vi "Initialize.vi"(8 "Error In":errorcluster, 11 "libssh2lv Shared Library":path=path "") -> (0 "Error Out":errorcluster, 3 "SSH":refnum<class "SSH.lvclass">)   [LabVIEW 2021, in "Field_RnD_Services_LIBSSH2_Toolkit.lvlib" / "SSH.lvclass"]
doc: "Initialize the underlying libssh2 library. This must be called, or executed, before using any other VIs in this toolkit. This typically initializes the cryptography library (OpenSSL), which is statically compiled with the libssh2lv shared library."
uses:
  220524-VNA RP FLAT.llb/SSH.lvclass
  220524-VNA RP FLAT.llb/SSH.lvclass/SSH.ctl
  220524-VNA RP FLAT.llb/Field_RnD_Services_LIBSSH2_Toolkit.lvlib
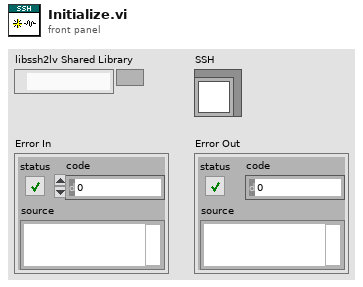
[diagram p1: front panel]
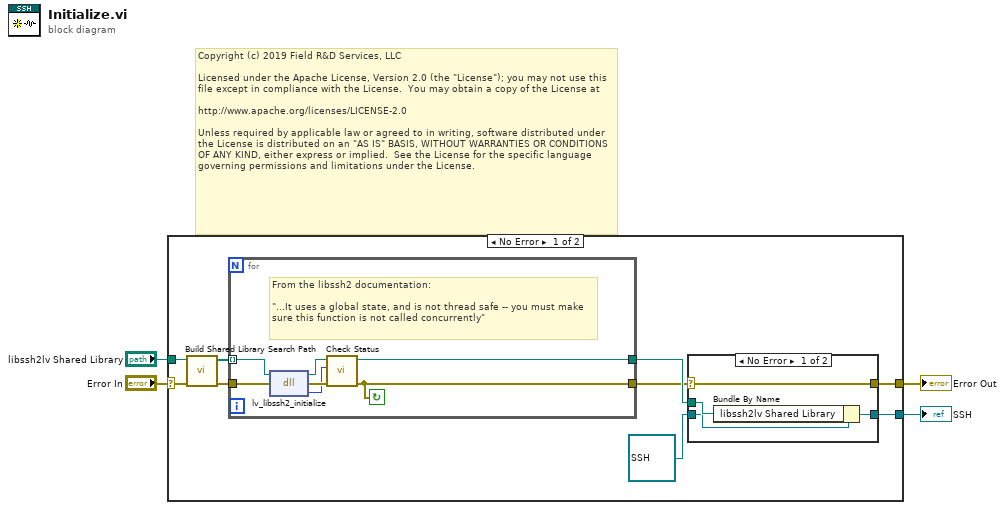
[diagram p0: block diagram]
diagram:
  # "Copyright (c) 2019 Field R&D Services, LLC\n\nLicensed under the Apache License, Version 2.0 (the \"License\"); you may not use this file except in compliance with the License.  You may obtain a copy of the License at\n\nhttp://www.apache.org/licenses/LICENSE-2.0\n\nUnless required by applicable law or agreed to in writing, software distributed under the License is distributed on an \"AS IS\" BASIS, WITHOUT WARRANTIES OR CONDITIONS OF ANY KIND, either express or implied.  See the License for the specific language governing permissions and limitations under the License."
  n1 = case shown="No Error" "Error In" {
    selector: "Error In" -> [w13 w27]
    tunnel: "libssh2lv Shared Library" -> [w12 _]
    tunnel: [w6 w27] -> w2
    tunnel: [w8 _] -> w1
    frame No Error {
      n2 = call "Build Shared Library Search Path.vi"("Error In"=w13, "libssh2lv Shared Library"=w12) -> ("Error Out"=w10:errorcluster, "Search Path"=w11:path[])  [unwired: 8 in]
      n3 = for {
        tunnel: w11 -> [w23] mode=indexing
        tunnel: w10 -> [w24]
        tunnel: [w26] -> w9
        tunnel: [w25] -> w7
        stop <- w25 continue-if-true
        # "From the libssh2 documentation:\n\n\"...It uses a global state, and is not thread safe -- you must make sure this function is not called concurrently\""
        n4 = dll-call lib="libssh2lv.*" fn="lv_libssh2_initialize"(path in=w23, error in=w24) -> (path out=w21:path, error out=w22:errorcluster, "return type"=w20:i32)  [unwired: 1 in]
        n5 = call "Check Status.vi"("Error In"=w22, "Status"=w20, "libssh2lv Shared Library In"=w21) -> ("Error Out"=w25:errorcluster, "libssh2lv Shared Library Out"=w26:path)  [unwired: 7 in]
      }
      n6 = case shown="No Error" w7 {
        selector: w7 -> [w15 w19]
        tunnel: w9 -> [w17 _]
        tunnel: [w16 w18] -> w8
        tunnel: [w15 w19] -> w6
        tunnel: refnum<class "SSH.lvclass"> refnum ("Toolkit.lvlib:SSH.lvclass") -> [w14 w18]
        frame No Error {
          n7 = Bundle By Name(cluster=w14, "libssh2lv Shared Library"=w17) -> (w16:refnum<class "SSH.lvclass">)
        }
        frame Error {
        }
      }
    }
    frame Error {
    }
  }
  "Error Out" <- w2
  "SSH" <- w1
